vi "From Pythonic - Tuple.vi"(4 "Pythonic Value":string) -> (1 "Tuple":string[](array[string]))   [LabVIEW 2012, in "OPI.lvclass"]
doc: "Convert pythonic values into LabVIEW data. This method can be helpfull to convert elements of tuples or dictionaries.\n\nReturn a 1D string array representing a tuple. Each index holds a pythonic value. Use indexing and the converter again on those values to convert them to LabVIEW data."
uses:
  OPI.lvclass
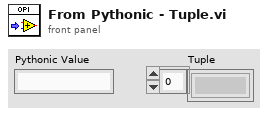
[diagram p1: front panel]
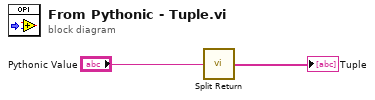
[diagram p0: block diagram]
diagram:
  n1 = call "Split Return.vi"("Return Value"="Pythonic Value") -> ("Split String"=→"Tuple":string[])
